vi "TCP_Client+命令.vi"() -> ()   [LabVIEW 2023]
uses:
  <vilib>/measure/NI_MABase.lvlib
panel:
  in  "信号类型":T1(ring)
  in  "方波占空比 (%)":dbl=50.0 caption="方波占空比(%)" format="%0.2f"
  in  "频率":dbl=10.0 format="%0.2p"
  in  "幅值":dbl=1.0 format="%0.2p"
  in  "参数发送":bool
  out "接收指示灯":bool
  in  "服务器IP":string
  out "文件传输进度":dbl(slide) scale=0.0..100.0
  in  "文件":bool
  in  "发送文件处理（打开:0）":T2(ring)
  in  "?":path
  in  "停止":bool
  in  "停止按钮":bool
  in  "消息发送":bool
  in  "发送字符串":string
  out "信息内容":string
  in  "停止":bool
  out "校验码":string
  out "接收时间":string
  out "文件内容":string
  out "文件字节数":string
  in  "接收文件处理（打开:0）":T2(ring)
  out "接收时间":string
  in  "服务器端口":dbl=7779.0
  # "TCP_Client"
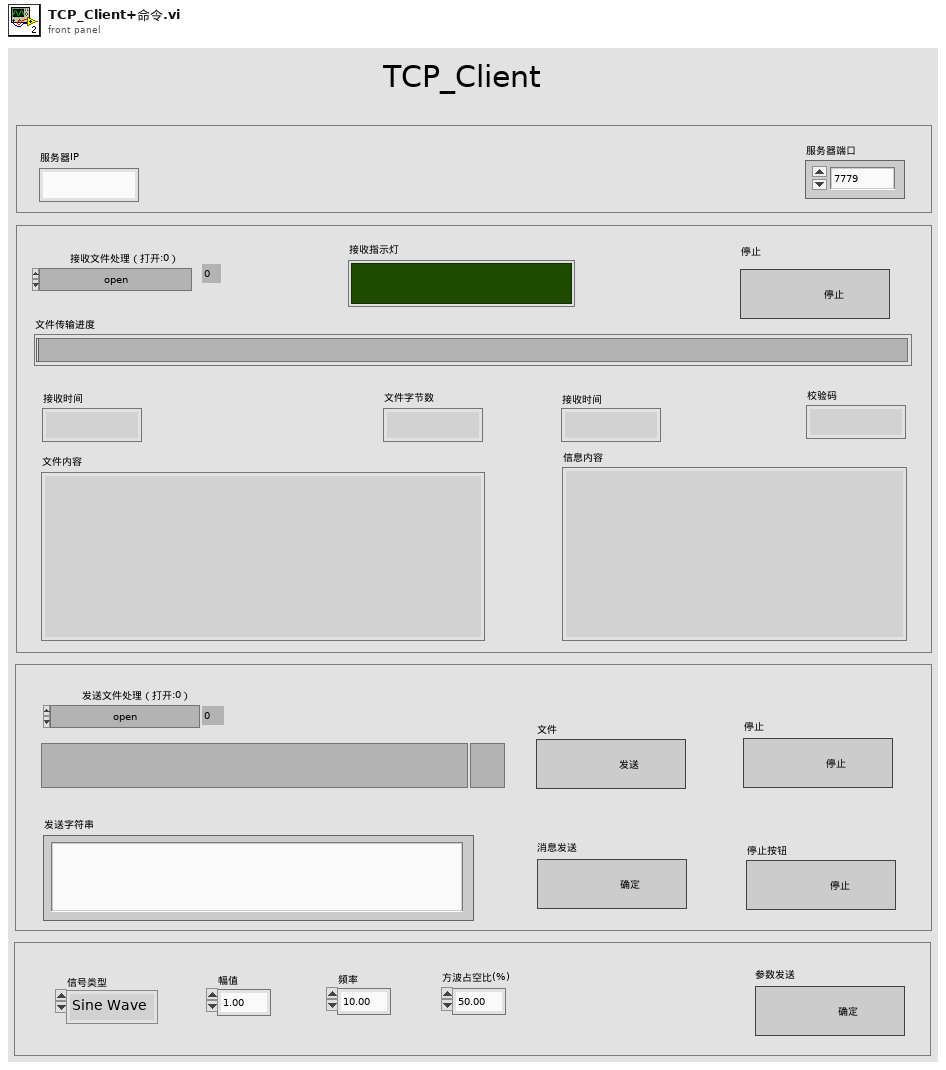
[diagram p1: front panel]
types:
  T1 = enum16{"Sine Wave", "Triangle Wave", "Square Wave", "Sawtooth Wave"}
  T2 = enum16{"open", "open or create", "create or replace", "create", "open (read only)"}
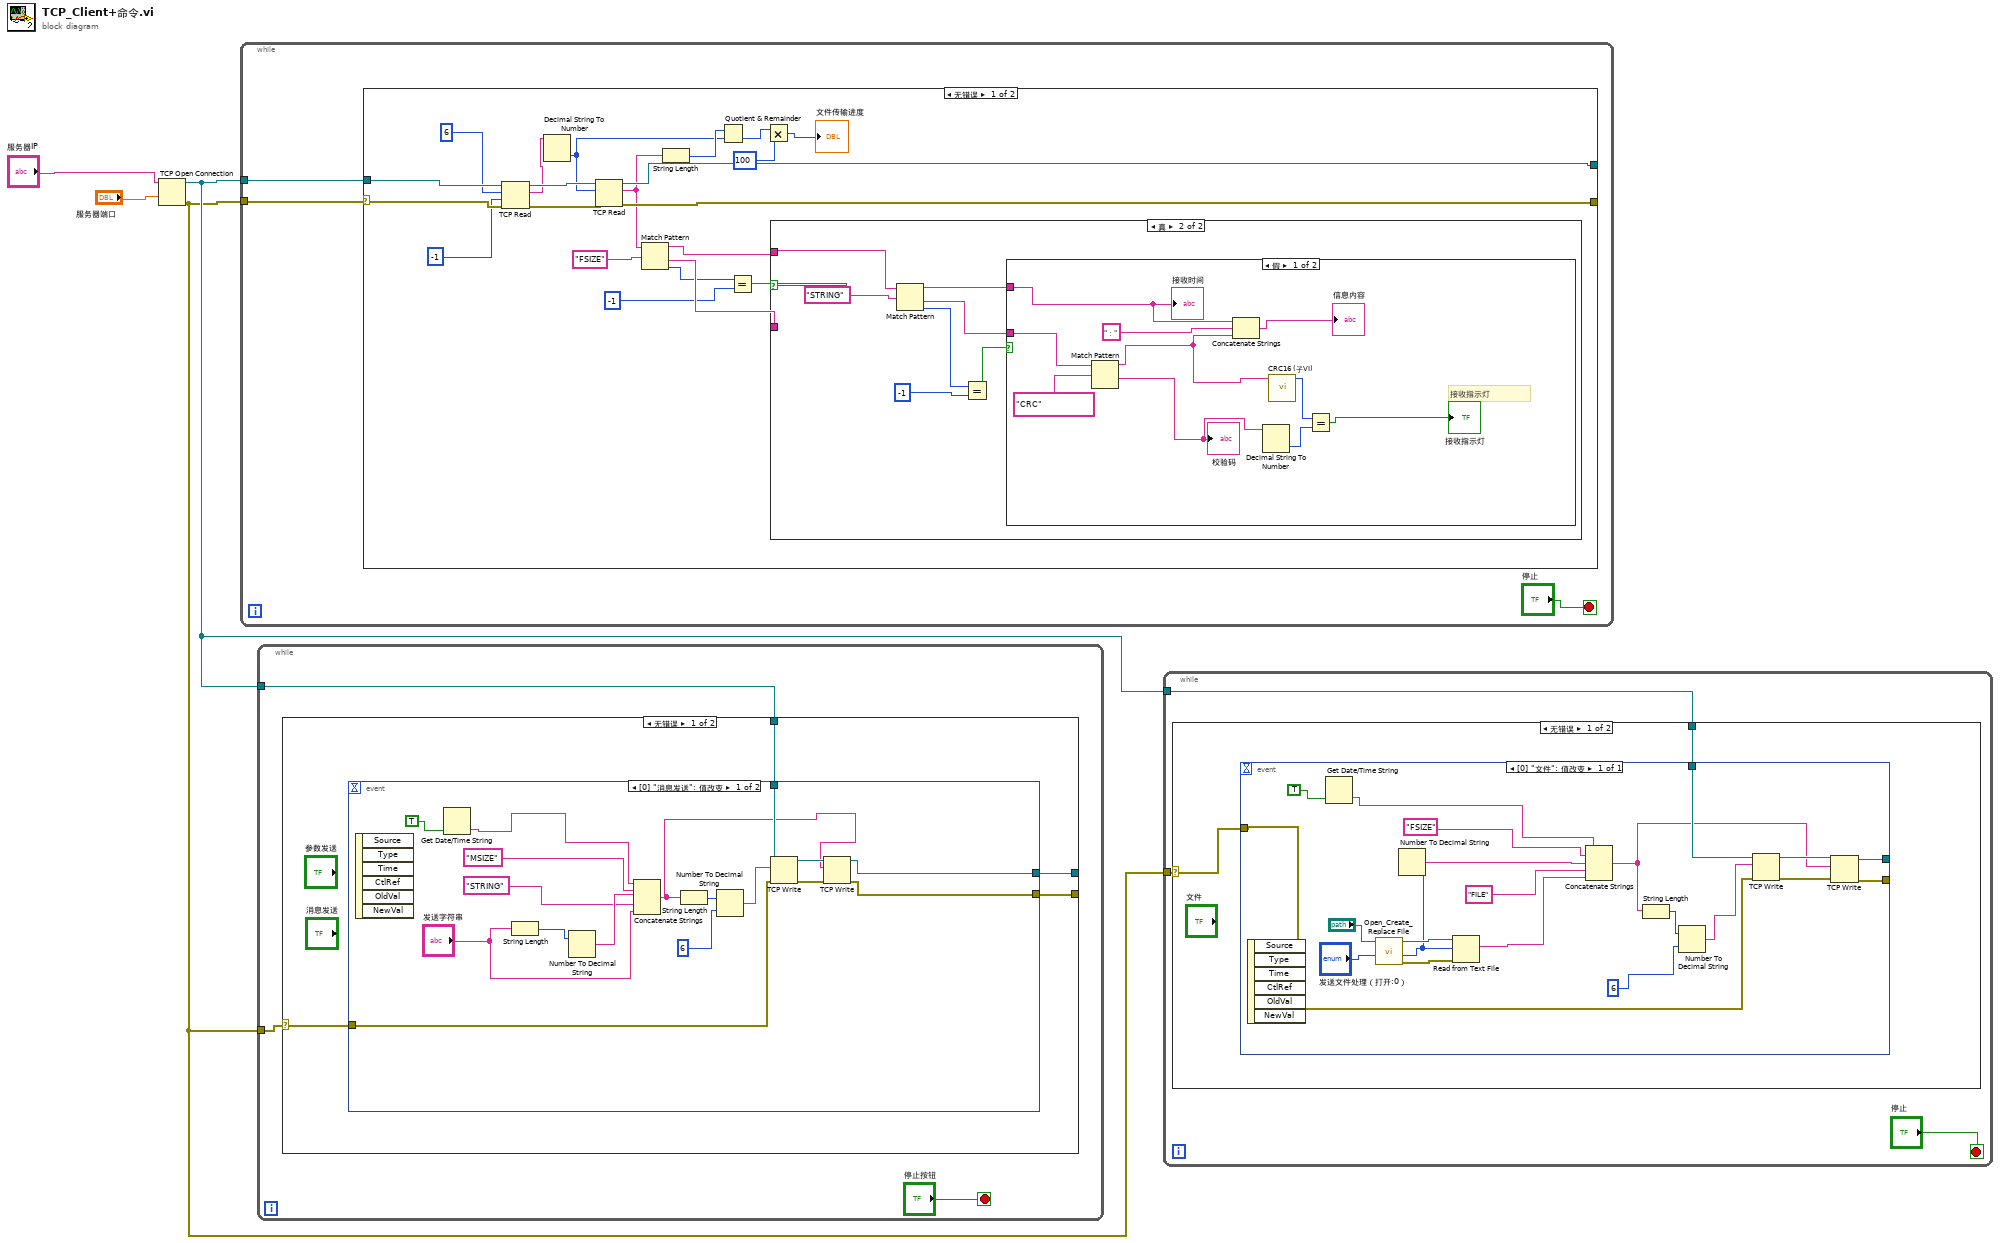
[diagram p0: block diagram]
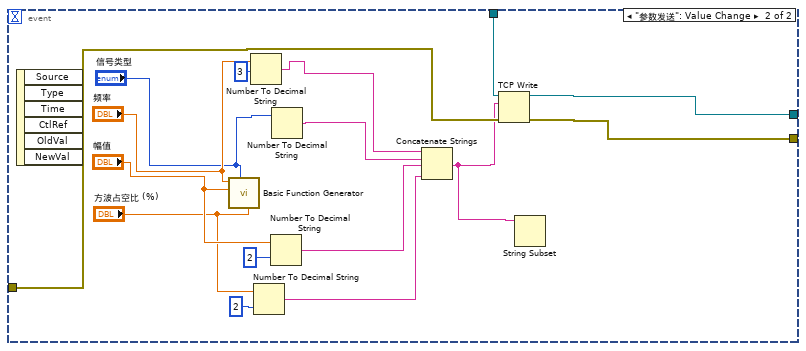
[diagram p3: hidden frame]
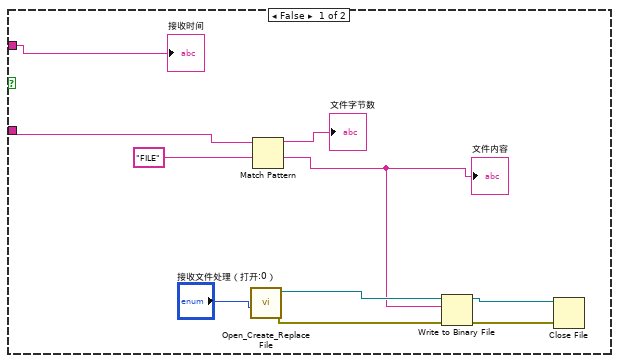
[diagram p5: hidden frame]
diagram:
  n1 = TCP Open Connection(address="服务器IP", remote port or service name="服务器端口") -> (connection ID=w3:refnum<k5>, error out=w2:errorcluster)  [unwired: 3 in]
  n2 = while {
    tunnel: w2 -> [w7]
    tunnel: w3 -> [w6]
    stop <- "停止" stop-if-true
    n3 = case shown="无错误" w7 {
      selector: w7 -> [w21 w56]
      tunnel: w6 -> [w22 w57]
      tunnel: [w17 w56] -> _
      tunnel: [w16 w57] -> _
      frame No Error {
        n4 = TCP Read(connection ID=w22, bytes to read=i16 6, error in (no error)=w21, 9:-1) -> (connection ID out=w19:refnum<k5>, data out=w14:string, error out=w18:errorcluster)  [unwired: 1 in]
        n5 = Decimal String To Number(string=w14) -> (number=w9:i32)  [unwired: 2 in, 1 out]
        n6 = TCP Read(connection ID=w19, bytes to read=w9, error in (no error)=w18) -> (connection ID out=w16:refnum<k5>, data out=w8:string, error out=w17:errorcluster)  [unwired: 2 in]
        n7 = Match Pattern(string=w8, regular expression="FSIZE") -> (before substring=w28:string, after substring=w27:string, offset past match=w25:i32)  [unwired: 1 in, 1 out]
        n8 = String Length(string=w8) -> (length=w13:i32)
        n9 = Quotient & Remainder(x=w13, y=w9) -> (floor(x/y)=w12:i32)  [unwired: 1 out]
        n10 = Equal?(x=w25, y=-1) -> (x = y?=w26:bool)
        n11 = Multiply(x=w12, y=100) -> (x*y=→"文件传输进度":i32)
        n12 = case shown="真" w26 {
          tunnel: w27 -> [w36 _]
          tunnel: w28 -> [w30 w44]
          frame False {
            n13 = call <vilib>:"Open_Create_Replace File.vi"("function (open:0)"="接收文件处理（打开:0）") -> ("error out"=w33:errorcluster, "refnum"=w34:refnum<file>)  [unwired: 7 in, 2 out]
            n14 = Match Pattern(string=w36, regular expression="FILE") -> (before substring=→"文件字节数":string, after substring=w29:string)  [unwired: 1 in, 2 out]
            "文件内容" <- w29
            n15 = Write to Binary File(file (use dialog)=w34, data=w29, error in=w33) -> (refnum out=w32:refnum<file>, error out=w31:errorcluster)  [unwired: 3 in, 1 out]
            n16 = Close File(refnum=w32, error in=w31) -> ()  [unwired: 2 out]
            "接收时间" <- w30
          }
          frame True {
            n17 = Match Pattern(string=w44, regular expression="STRING") -> (before substring=w39:string, after substring=w40:string, offset past match=w43:i32)  [unwired: 1 in, 1 out]
            n18 = Equal?(x=w43, y=-1) -> (x = y?=w41:bool)
            n19 = case shown="假" w41 {
              tunnel: w40 -> [w54 _]
              tunnel: w39 -> [w49 _]
              frame False {
                # "接收指示灯"
                n20 = Match Pattern(string=w54, regular expression="CRC") -> (before substring=w47:string, after substring=w53:string)  [unwired: 1 in, 2 out]
                "校验码" <- w53
                n21 = Concatenate Strings(w49, "：", w47) -> (→"信息内容":string)
                n22 = Decimal String To Number(string=w53) -> (number=w50:i32)  [unwired: 2 in, 1 out]
                n23 = call "CRC16 (子VI).vi"("字符串"=w47) -> ("数值"=w52:u16)  [unwired: 10 in]
                n24 = Equal?(x=w52, y=w50) -> (x = y?=→"接收指示灯":bool)
                "接收时间" <- w49
              }
              frame True {
              }
            }
          }
        }
      }
      frame Error {
      }
    }
  }
  n25 = while {
    tunnel: w2 -> [w60]
    tunnel: w3 -> [w59]
    stop <- "停止按钮" stop-if-true
    n26 = case shown="无错误" w60 {
      selector: w60 -> [w64 w99]
      tunnel: w59 -> [w63 w98]
      tunnel: [w62 w99] -> _
      tunnel: [w61 w98] -> _
      frame No Error {
        n27 = event shown="[0] \"消息发送\": 值改变" {
          selector: _ -> [_ _]
          dyn-events: _ -> [_ _]
          timeout: _ -> [_ _]
          tunnel: w64 -> [w81 w86]
          tunnel: w63 -> [w73 w87]
          tunnel: [w72 w84] -> w62
          tunnel: [w71 w85] -> w61
          event "消息发送": Value Change {
            n28 = event-data() -> ()  [unwired: 1 in, 6 out]
            n29 = Get Date/Time String(want seconds? (F)=TRUE) -> (time string=w67:string)  [unwired: 2 in, 1 out]
            n30 = String Length(string="发送字符串") -> (length=w79:i32)
            n31 = Number To Decimal String(number=w79) -> (decimal integer string=w78:string)  [unwired: 1 in]
            n32 = Concatenate Strings(w67, "MSIZE", w78, "STRING", "发送字符串") -> (w65:string)
            n33 = String Length(string=w65) -> (length=w70:i32)
            n34 = Number To Decimal String(number=w70, width (-)=6) -> (decimal integer string=w69:string)
            n35 = TCP Write(connection ID=w73, data in=w69, error in (no error)=w81) -> (connection ID out=w75:refnum<k5>, error out=w74:errorcluster)  [unwired: 1 in, 1 out]
            n36 = TCP Write(connection ID=w75, data in=w65, error in (no error)=w74) -> (connection ID out=w71:refnum<k5>, error out=w72:errorcluster)  [unwired: 1 in, 1 out]
          }
          event "参数发送": Value Change {
            n37 = event-data() -> ()  [unwired: 1 in, 6 out]
            n38 = call <vilib>:"Basic Function Generator.vi"("square wave duty cycle (%)"="方波占空比 (%)", "signal type"="信号类型", "amplitude"="幅值", "frequency"="频率") -> ()  [unwired: 5 in, 3 out]
            n39 = Number To Decimal String(number="频率", width (-)=3) -> (decimal integer string=w97:string)
            n40 = Number To Decimal String(number="方波占空比 (%)", width (-)=2) -> (decimal integer string=w88:string)
            n41 = Number To Decimal String(number="幅值", width (-)=2) -> (decimal integer string=w89:string)
            n42 = Number To Decimal String(number="信号类型") -> (decimal integer string=w96:string)  [unwired: 1 in]
            n43 = Concatenate Strings(w97, w96, w89, w88) -> (w83:string)
            n44 = TCP Write(connection ID=w87, data in=w83, error in (no error)=w86) -> (connection ID out=w85:refnum<k5>, error out=w84:errorcluster)  [unwired: 1 in, 1 out]
            n45 = String Subset(string=w83) -> ()  [unwired: 2 in, 1 out]
          }
        }
      }
      frame Error {
      }
    }
  }
  n46 = while {
    tunnel: w2 -> [w102]
    tunnel: w3 -> [w101]
    stop <- "停止" stop-if-true
    n47 = case shown="无错误" w102 {
      selector: w102 -> [w104 _]
      tunnel: w101 -> [w103 _]
      frame No Error {
        n48 = event shown="[0] \"文件\": 值改变" {
          selector: _ -> [_]
          dyn-events: _ -> [_]
          timeout: _ -> [_]
          tunnel: w104 -> [w113]
          tunnel: w103 -> [w116]
          tunnel: [w111] -> _
          tunnel: [w110] -> _
          event "文件": Value Change {
            n49 = event-data() -> ()  [unwired: 1 in, 6 out]
            n50 = Get Date/Time String(want seconds? (F)=TRUE) -> (time string=w108:string)  [unwired: 2 in, 1 out]
            n51 = call <vilib>:"Open_Create_Replace File.vi"("function (open:0)"="发送文件处理（打开:0）", "file path"="?") -> ("error out"=w123:errorcluster, "file size (bytes)"=w121:i32, "refnum"=w122:refnum<file>)  [unwired: 6 in, 1 out]
            n52 = Number To Decimal String(number=w121) -> (decimal integer string=w118:string)  [unwired: 1 in]
            n53 = Read from Text File(file (use dialog)=w122, count=w121, error in=w123) -> (text=w120:string)  [unwired: 1 in, 3 out]
            n54 = Concatenate Strings(w108, "FSIZE", w118, "FILE", w120) -> (w114:string)
            n55 = String Length(string=w114) -> (length=w107:i32)
            n56 = Number To Decimal String(number=w107, width (-)=6) -> (decimal integer string=w105:string)
            n57 = TCP Write(connection ID=w116, data in=w105, error in (no error)=w113) -> (connection ID out=w115:refnum<k5>, error out=w112:errorcluster)  [unwired: 1 in, 1 out]
            n58 = TCP Write(connection ID=w115, data in=w114, error in (no error)=w112) -> (connection ID out=w111:refnum<k5>, error out=w110:errorcluster)  [unwired: 1 in, 1 out]
          }
        }
      }
      frame Error {
      }
    }
  }
